vi "Reciprocal.vi"   [LabVIEW 2019, in "xy_utilities.lvlib"]
doc: "Take the reciprocal of <b>XY-data</b>'s y array.\n\nWire data to the data input to determine the polymorphic instance to use or manually select the instance."
uses:
  xy_utilities.lvlib
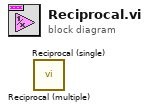
[diagram p0: block diagram]
diagram:
  n1 = call "Reciprocal (multiple).vi"() -> ()  [unwired: 10 in, 2 out]
  n2 = call "Reciprocal (single).vi"() -> ()  [unwired: 10 in, 2 out]
